vi "Configure Under Voltage Limit.vi"(7 "Slave Address":i32=-1 min=-1 max=30 step=1, 8 "error":errorcluster, 10 "UVL Level":dbl format="%.4f", 11 "VISA":refnum<visa-resource-name>) -> (0 "error out":errorcluster, 3 "VISA out":refnum<visa-resource-name>)   [LabVIEW 2025, in "TDK-Lambda GEN LAN Series.lvlib"]
doc: "Configure the Under-Voltage Limit (UVL). The power supply voltage may be set no lower than approx 5% above this limit. \n\nThis is not an output protection; there is no fault if the actual output falls below this limit"
uses:
  <userlib>/TDK-Lambda GEN LAN Series/TDK-Lambda GEN LAN Series.lvlib
panel:
  # "TDK-Lambda Genesys \n LAN\n  DC Power Supplies"
  # "Set the Under-Voltage \nLimit  (UVL)"
  # "(c) 2019 TDK-Lambda.  ALL RIGHTS RESERVED."
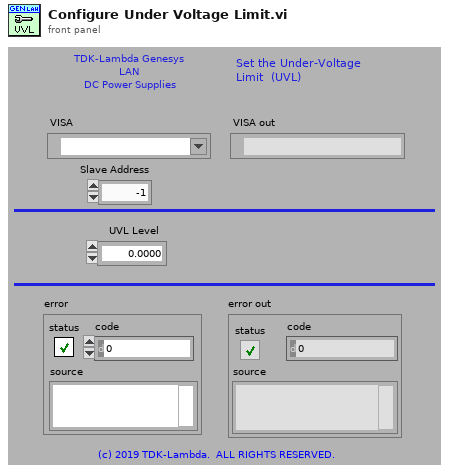
[diagram p1: front panel]
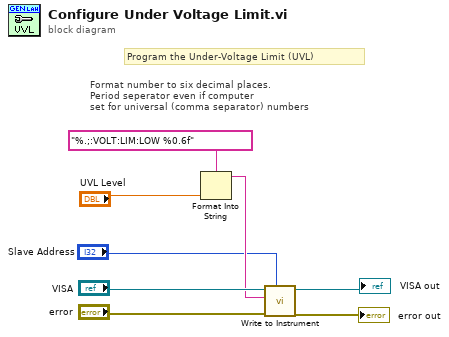
[diagram p0: block diagram]
diagram:
  # "Format number to six decimal places.\nPeriod seperator even if computer \nset for universal (comma separator) numbers"
  # "Program the Under-Voltage Limit (UVL)"
  n1 = Format Into String(format string="%.;:VOLT:LIM:LOW %0.6f", "UVL Level") -> (resulting string=w4:string)  [unwired: 2 in, 1 out]
  n2 = call <userlib>:"Write to Instrument.vi"("Slave Address"="Slave Address", "error"="error", "Command"=w4, "VISA"="VISA") -> ("error out"=→"error out":errorcluster, "VISA out"=→"VISA out":refnum<visa-resource-name>)  [unwired: 6 in]
